vi "m-q.vi"(0 "x1":dbl, 3 "x2":dbl, 4 "y1":dbl, 5 "y2":dbl) -> (1 "q":dbl, 2 "m":dbl)   [LabVIEW 2011]
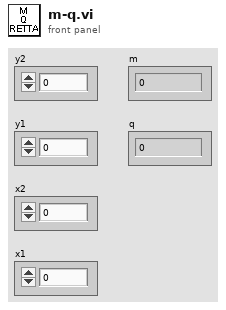
[diagram p1: front panel]
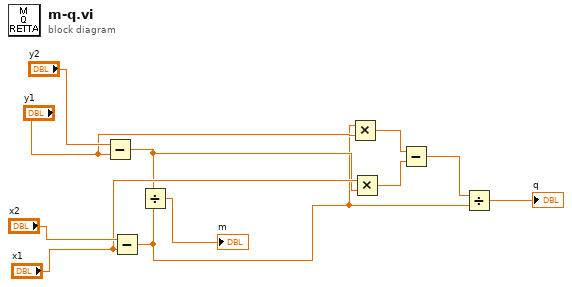
[diagram p0: block diagram]
diagram:
  n1 = Subtract(x="y2", y="y1") -> (x-y=w4:dbl)
  n2 = Subtract(x="x2", y="x1") -> (x-y=w1:dbl)
  n3 = Divide(x=w4, y=w1) -> (x/y=→"m":dbl)
  n4 = Multiply(x=w1, y="y1") -> (x*y=w6:dbl)
  n5 = Multiply(x="x1", y=w4) -> (x*y=w3:dbl)
  n6 = Subtract(x=w6, y=w3) -> (x-y=w2:dbl)
  n7 = Divide(x=w2, y=w1) -> (x/y=→"q":dbl)
